vi "SplitStatus.vi"(9 "Index":i32, 11 "Input String":string) -> (3 "Out":string)   [LabVIEW 2020]
panel:
  out "All":string[](array[string])
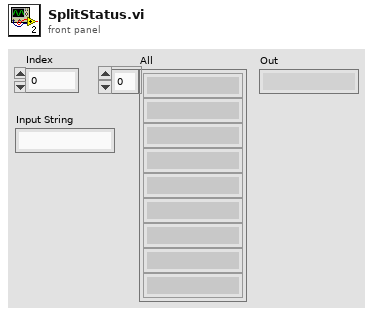
[diagram p1: front panel]
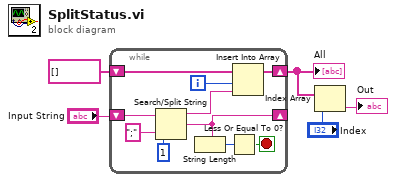
[diagram p0: block diagram]
diagram:
  n1 = while {
    shift-right: [w12] -> _
    shift-left: "Input String" -> [w14]
    shift-right: [w7] -> w4
    shift-left: string[] [] -> [w8]
    i -> [w6]
    stop <- w10 stop-if-true
    n2 = Search/Split String(string=w14, search string/char (-)=";", offset (0)=1) -> (substring before match=w9:string, match + rest of string=w12:string)  [unwired: 1 out]
    n3 = String Length(string=w12) -> (length=w11:i32)
    n4 = Less Or Equal To 0?(x=w11) -> (x <= 0?=w10:bool)
    n5 = Insert Into Array(array=w8, index=w6, new element=w9) -> (w7:string[])
  }
  "All" <- w4
  n6 = Index Array(array=w4, index="Index") -> (element=→"Out":string)
